vi "Poll.GetTreeSelection.vi"(8 "error in (no error)":errorcluster, 10 "Input Channels":variant, 11 ".NET Refnum in":refnum<k24>) -> (0 "error out":errorcluster, 3 "Refs":T1[](array[typedef]) format="%.0x")   [LabVIEW 2017, in "OPC UA Client System Explorer.lvlib"]
uses:
  OPC UA Client System Explorer.lvlib
  NationalInstruments.VeriStand.SystemStorageUI
  <vilib>/NI Veristand/Custom Device API/Custom Device Item Ref.ctl
  NationalInstruments.VeriStand.SystemStorage
  <vilib>/NI VeriStand/Custom Device API/Custom Device API.lvlib
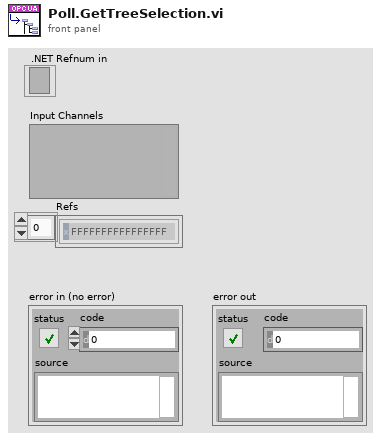
[diagram p1: front panel]
types:
  T1 = typedef "Custom Device API.lvlib/Custom Device Item Ref.ctl" = u64
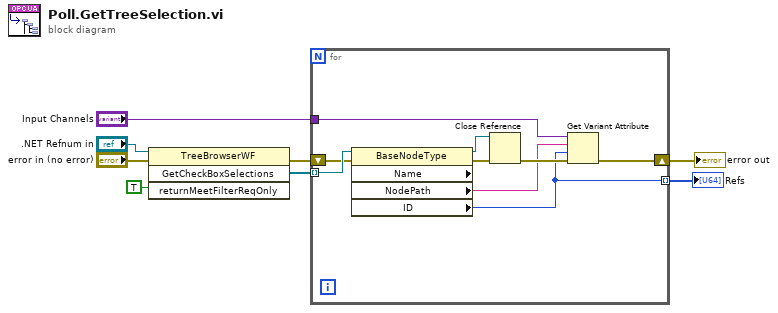
[diagram p0: block diagram]
diagram:
  n1 = invoke class="TreeBrowserWF" method="GetCheckBoxSelections"(reference=".NET Refnum in", error in="error in (no error)", "returnMeetFilterReqOnly"=TRUE) -> (error out=w6:errorcluster, "GetCheckBoxSelections"=w5:refnum<k24>[])  [unwired: 1 in, 2 out]
  n2 = for {
    tunnel: w5 -> [w17] mode=indexing
    shift-right: [w15] -> w7
    shift-left: w6 -> [w16]
    tunnel: [w9] -> w1 mode=indexing
    tunnel: "Input Channels" -> [w14]
    n3 = property class="BaseNodeType" props=["Name", "NodePath", "ID"](reference=w17, error in=w16) -> (reference out=w11:refnum<k24>, error out=w13:errorcluster, "NodePath"=w10:string, "ID"=w9:u64)  [unwired: 1 out]
    n4 = Close Reference(reference=w11, error in (no error)=w13) -> (error out=w12:errorcluster)
    n5 = Get Variant Attribute(Variant=w14, name=w10, default value (empty Variant)=w9, error in=w12) -> (error out=w15:errorcluster)  [unwired: 3 out]
  }
  "error out" <- w7
  "Refs" <- w1
